vi "freq file -- file type selector.vi"(7 "folder kind":T1=enum."9w", 11 "Sweep folder path":path=path "\\\\rus-one\\newdata/data/Ultrasound/Experiment/ProbeTest/Probe10/Hg1201-4-C199-80K-1/Sweep1") -> (0 "file name regular expression":string, 2 "folder path":path, 3 "OK":bool)   [LabVIEW 2015]
uses:
  freq file -- file select folder control.ctl
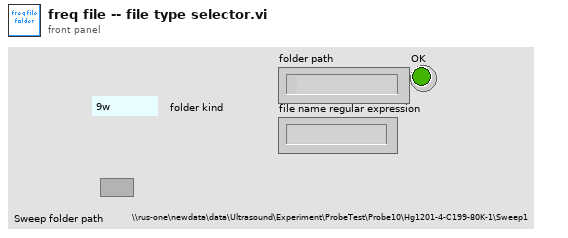
[diagram p1: front panel]
types:
  T1 = typedef "freq file -- file select folder control.ctl" = enum16{"monitor", "9w"}
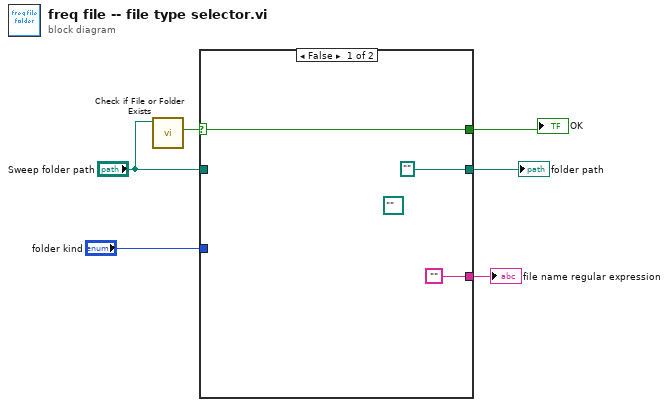
[diagram p0: block diagram]
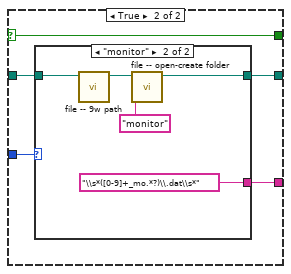
[diagram p2: hidden frame]
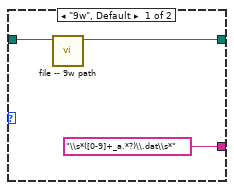
[diagram p3: hidden frame]
diagram:
  n1 = call <vilib>:"Check if File or Folder Exists.vi"("path"="Sweep folder path") -> ("file or folder exists?"=w2:bool)  [unwired: 8 in, 2 out]
  n2 = case shown="False" w2 {
    selector: w2 -> [w9 w10]
    tunnel: "folder kind" -> [_ w14]
    tunnel: [path "" w13] -> w5
    tunnel: ["" w12] -> w4
    tunnel: "Sweep folder path" -> [_ w11]
    tunnel: [w9 w10] -> w1
    frame False {
      (unwired) path "" ("folder path out")
    }
    frame True {
      n3 = case shown="\"monitor\"" w14 {
        tunnel: w11 -> [w17 w22]
        tunnel: [w16 w18] -> w13
        tunnel: ["\\s*([0-9]+_a.*?)\\.dat\\s*" ("regular expression") "\\s*([0-9]+_mo.*?)\\.dat\\s*" ("regular expression")] -> w12
        frame "9w", Default {
          n4 = call "file -- 9w path.vi"("sweep folder"=w17) -> ("9w path"=w16:path)  [unwired: 10 in]
        }
        frame "monitor" {
          n5 = call "file -- 9w path.vi"("sweep folder"=w22) -> ("9w path"=w19:path)  [unwired: 10 in]
          n6 = call "file -- open-create folder.vi"("folder name"="monitor" ("name or relative path"), "base path"=w19) -> ("folder path out"=w18:path)  [unwired: 9 in]
        }
      }
    }
  }
  "folder path" <- w5
  "file name regular expression" <- w4
  "OK" <- w1
